vi "Send Exposure Time.vi"(8 "error in":errorcluster, 10 "Exposure Time (ms)":dbl=200.0 min=0.06 max=200.0 step=0.01) -> (0 "error out":errorcluster, 1 "Send Error":bool, 2 "Time Set":bool)   [LabVIEW 2009]
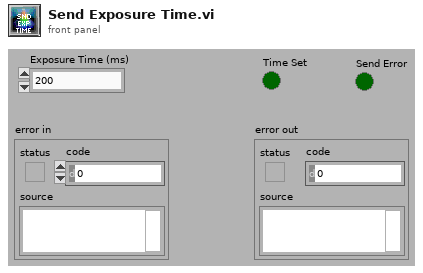
[diagram p1: front panel]
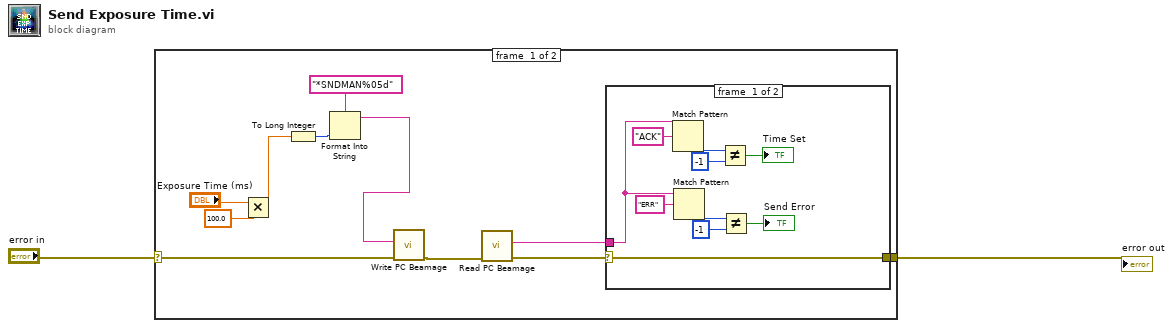
[diagram p0: block diagram]
diagram:
  n1 = case shown="No Error" "error in" {
    selector: "error in" -> [w13 w25]
    tunnel: [w9 w25] -> w1
    frame #0 {
      n2 = Multiply(x="Exposure Time (ms)", y=100.0) -> (x*y=w4:dbl)
      n3 = To Long Integer(number=w4) -> (32bit integer=w3:i32)
      n4 = Format Into String(format string="*SNDMAN%05d" ("command"), w3) -> (resulting string=w8:string)  [unwired: 2 in, 1 out]
      n5 = call "Write PC Beamage.vi"("error in"=w13, "command"=w8) -> ("error out"=w12:errorcluster)  [unwired: 9 in]
      n6 = call "Read PC Beamage.vi"("error in"=w12) -> ("error out"=w11:errorcluster, "Reply"=w10:string)  [unwired: 9 in]
      n7 = case shown="No Error" w11 {
        selector: w11 -> [w14 w24]
        tunnel: w10 -> [w15 _]
        tunnel: [w14 w24] -> w9
        frame #0 {
          n8 = Match Pattern(string=w15, regular expression="ACK") -> (offset past match=w22:i32)  [unwired: 1 in, 3 out]
          n9 = Match Pattern(string=w15, regular expression="ERR") -> (offset past match=w18:i32)  [unwired: 1 in, 3 out]
          n10 = Not Equal?(x=w22, y=-1) -> (x != y?=→"Time Set":bool)
          n11 = Not Equal?(x=w18, y=-1) -> (x != y?=→"Send Error":bool)
        }
        frame #1 {
        }
      }
    }
    frame #1 {
    }
  }
  "error out" <- w1
